vi "EminemBegin.vi"(6 "error in (no error)":errorcluster) -> (0 "error out":errorcluster)   [LabVIEW 2023]
doc: "Opens motors and sensors for Eminem subassembly\nInputs:\n--Error in--error type\nOutputs:\n--Error out--error type"
uses:
  <vilib>/Rock Robotics/WPI/ThirdParty/REV Robotics/REVLib/Typedef/Spark MAX Motor Type.ctl
  <vilib>/Rock Robotics/WPI/ThirdParty/REV Robotics/REVLib/Typedef/Spark MAX Idle Mode.ctl
  <vilib>/Rock Robotics/SystemInterfaces/DIO/FPGA_DIOChannel.ctl
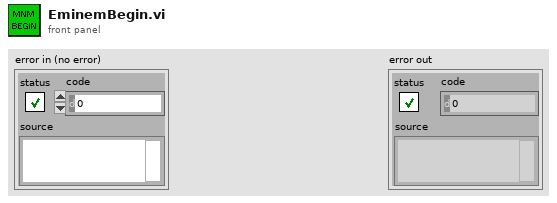
[diagram p1: front panel]
types:
  T1 = typedef "Spark MAX Idle Mode.ctl" = enum16{"Coast", "Brake"}
  T2 = typedef "Spark MAX Motor Type.ctl" = enum16{"Brushed", "Brushless"}
  T3 = typedef "WPI_MotorControlDeviceRef.ctl" = cluster{"DeviceStatus":errorcluster, "Type":T4, "PWM":cluster{"PWM Channel":T5, "DeadBand":T6}, "CAN":cluster{"Device Number":u8, "SetOutput VI Ref":variant, "GetOutput VI Ref":variant, "Enable VI Ref":variant, "Disable VI Ref":variant, "Data":variant}, "Invert":bool, "DIO PWM":cluster{"PWM \"Enable\" Channel":T5, "DIOChannel":T7, "PWM Rate":dbl}}
  T4 = typedef "WPI_MotorControlType.ctl" = enum16{"PWM", "CAN", "DIO PWM"}
  T5 = typedef "FPGA_DIOPWMChannel.ctl" = enum8{"PWM 0", "PWM 1", "PWM 2", "PWM 3", "PWM 4", "PWM 5", "PWM 6", "PWM 7", "PWM 8", "PWM 9", "PWM MXP 0", "PWM MXP 1", "PWM MXP 2", "PWM MXP 3", "PWM MXP 4", "PWM MXP 5", "PWM MXP 6", "PWM MXP 7", "PWM MXP 8", "PWM MXP 9", "Invalid"}
  T6 = typedef "WPI_PWMDeadband.ctl" = cluster{"Name":string, "maxPositivePwm":i32, "minPositivePwm":i32, "centerPwm":i32, "maxNegativePwm":i32, "minNegativePwm":i32, "angularRange":u16}
  T7 = typedef "FPGA_DIOChannel.ctl" = enum8{"DIO 0", "DIO 1", "DIO 2", "DIO 3", "DIO 4", "DIO 5", "DIO 6", "DIO 7", "DIO 8", "DIO 9", "DIO MXP 0", "DIO MXP 1", "DIO MXP 2", "DIO MXP 3", "DIO MXP 4", "DIO MXP 5", "DIO MXP 6", "DIO MXP 7", "DIO MXP 8", "DIO MXP 9", "DIO MXP 10", "DIO MXP 11", "DIO MXP 12", "DIO MXP 13", "DIO MXP 14", "DIO MXP 15", "SPI Port CS1", "SPI Port CS2", "SPI Port CS3", "SPI Port MISO", "SPI Port MOSI", "Invalid"}
  T8 = typedef "WPI_DigitalInputDevRef.ctl" = cluster{"DevStatus":errorcluster, "DIO Channel":T7}
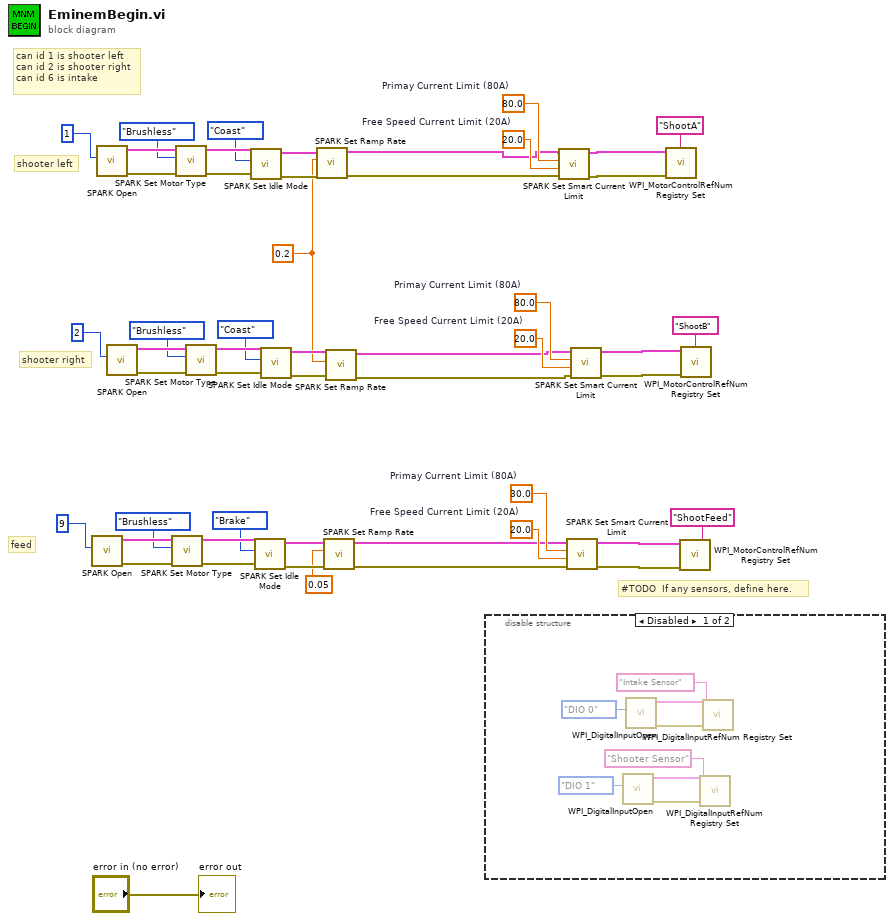
[diagram p0: block diagram]
diagram:
  w7 = 20.0  # Free Speed Current Limit (20A)
  w8 = 80.0  # Primay Current Limit (80A)
  w13 = 20.0  # Free Speed Current Limit (20A)
  w14 = 80.0  # Primay Current Limit (80A)
  w15 = 20.0  # Free Speed Current Limit (20A)
  w16 = 30.0  # Primay Current Limit (80A)
  w20 = 0.2
  # "#TODO  If any sensors, define here."
  # "feed"
  # "shooter right"
  # "shooter left"
  # "can id 1 is shooter left\ncan id 2 is shooter right\ncan id 6 is intake"
  n1 = call <vilib>:"SPARK Open.vi"("Device Number"=9) -> ("error out"=w30:errorcluster, "MotorControlDeviceRef"=w32:T3)  [unwired: 9 in]
  n2 = call <vilib>:"SPARK Open.vi"("Device Number"=1) -> ("error out"=w46:errorcluster, "MotorControlDeviceRef"=w48:T3)  [unwired: 9 in]
  n3 = call <vilib>:"SPARK Open.vi"("Device Number"=2) -> ("error out"=w38:errorcluster, "MotorControlDeviceRef"=w40:T3)  [unwired: 9 in]
  n4 = call <vilib>:"SPARK Set Motor Type.vi"("error in (no error)"=w30, "Motor Type"=Spark_MAX_Motor_Type."Brushless", "MotorControlDevRef"=w32) -> ("error out"=w29:errorcluster, "MotorControlDeviceRef"=w31:T3)  [unwired: 7 in]
  n5 = call <vilib>:"SPARK Set Motor Type.vi"("error in (no error)"=w46, "Motor Type"=Spark_MAX_Motor_Type."Brushless", "MotorControlDevRef"=w48) -> ("error out"=w45:errorcluster, "MotorControlDeviceRef"=w47:T3)  [unwired: 7 in]
  n6 = call <vilib>:"SPARK Set Motor Type.vi"("error in (no error)"=w38, "Motor Type"=Spark_MAX_Motor_Type."Brushless", "MotorControlDevRef"=w40) -> ("error out"=w37:errorcluster, "MotorControlDeviceRef"=w39:T3)  [unwired: 7 in]
  n7 = call <vilib>:"SPARK Set Idle Mode.vi"("error in (no error)"=w45, "Idle Mode"=Spark_MAX_Idle_Mode."Coast", "MotorControlDeviceRef in"=w47) -> ("error out"=w24:errorcluster, "MotorControlDeviceRef out"=w23:T3)  [unwired: 7 in]
  n8 = call <vilib>:"SPARK Set Idle Mode.vi"("error in (no error)"=w29, "Idle Mode"=Spark_MAX_Idle_Mode."Brake", "MotorControlDeviceRef in"=w31) -> ("error out"=w21:errorcluster, "MotorControlDeviceRef out"=w22:T3)  [unwired: 7 in]
  n9 = call <vilib>:"SPARK Set Idle Mode.vi"("error in (no error)"=w37, "Idle Mode"=Spark_MAX_Idle_Mode."Coast", "MotorControlDeviceRef in"=w39) -> ("error out"=w25:errorcluster, "MotorControlDeviceRef out"=w26:T3)  [unwired: 7 in]
  n10 = call <vilib>:"SPARK Set Ramp Rate.vi"("error in (no error)"=w24, "Seconds from neutral to full (0)"=w20, "MotorControlDeviceRef in"=w23) -> ("error out"=w5:errorcluster, "MotorControlDeviceRef"=w6:T3)  [unwired: 7 in]
  n11 = call <vilib>:"SPARK Set Ramp Rate.vi"("error in (no error)"=w21, "Seconds from neutral to full (0)"=0.05, "MotorControlDeviceRef in"=w22) -> ("error out"=w2:errorcluster, "MotorControlDeviceRef"=w1:T3)  [unwired: 7 in]
  n12 = call <vilib>:"SPARK Set Ramp Rate.vi"("error in (no error)"=w25, "Seconds from neutral to full (0)"=w20, "MotorControlDeviceRef in"=w26) -> ("error out"=w11:errorcluster, "MotorControlDeviceRef"=w12:T3)  [unwired: 7 in]
  n13 = disable-structure shown="Disabled" {
    frame Disabled {
      n14 = call <vilib>:"WPI_DigitalInputOpen.vi"("DIO Channel"=FPGA_DIOChannel."DIO 1") -> ("error out"=w54:errorcluster, "DigitalInputDevRef"=w53:T8)  [unwired: 9 in]
      n15 = call <vilib>:"WPI_DigitalInputOpen.vi"("DIO Channel"=FPGA_DIOChannel."DIO 0") -> ("error out"=w58:errorcluster, "DigitalInputDevRef"=w57:T8)  [unwired: 9 in]
      n16 = call <vilib>:"WPI_DigitalInputRefNum Registry Set.vi"("error in (no error)"=w54, "refnum name"="Shooter Sensor", "DigitalInputDevRef"=w53) -> ()  [unwired: 7 in, 2 out]
      n17 = call <vilib>:"WPI_DigitalInputRefNum Registry Set.vi"("error in (no error)"=w58, "refnum name"="Intake Sensor", "DigitalInputDevRef"=w57) -> ()  [unwired: 7 in, 2 out]
    }
    frame Enabled {
    }
  }
  n18 = call <vilib>:"SPARK Set Smart Current Limit.vi"("error in (no error)"=w5, "Free Speed Current Limit (20A)"=w7, "Primay Current Limit (80A)"=w8, "MotorControlDeviceRef in"=w6) -> ("error out"=w3:errorcluster, "MotorControlDeviceRef out"=w4:T3)  [unwired: 6 in]
  n19 = call <vilib>:"SPARK Set Smart Current Limit.vi"("error in (no error)"=w2, "Free Speed Current Limit (20A)"=w15, "Primay Current Limit (80A)"=w16, "MotorControlDeviceRef in"=w1) -> ("error out"=w17:errorcluster, "MotorControlDeviceRef out"=w18:T3)  [unwired: 6 in]
  n20 = call <vilib>:"SPARK Set Smart Current Limit.vi"("error in (no error)"=w11, "Free Speed Current Limit (20A)"=w13, "Primay Current Limit (80A)"=w14, "MotorControlDeviceRef in"=w12) -> ("error out"=w9:errorcluster, "MotorControlDeviceRef out"=w10:T3)  [unwired: 6 in]
  n21 = call <vilib>:"WPI_MotorControlRefNum Registry Set.vi"("error in (no error)"=w3, "refnum name"="ShootA", "MotorControlDevRef"=w4) -> ()  [unwired: 7 in, 2 out]
  n22 = call <vilib>:"WPI_MotorControlRefNum Registry Set.vi"("error in (no error)"=w17, "refnum name"="ShootFeed", "MotorControlDevRef"=w18) -> ()  [unwired: 7 in, 2 out]
  n23 = call <vilib>:"WPI_MotorControlRefNum Registry Set.vi"("error in (no error)"=w9, "refnum name"="ShootB", "MotorControlDevRef"=w10) -> ()  [unwired: 7 in, 2 out]
  "error out" <- "error in (no error)"
